vi "cblas ztrmm.vi"(0 "A":T2, 1 "B":T2, 3 "alpha":cdb=1.0+0.0i, 5 "order":T5=101 items=["CblasRowMajor"=101, "CblasColMajor"=102], 6 "transA":T6=111 items=["CblasNoTrans"=111, "CblasTrans"=112, "CblasConjTrans "=113], 7 "uplo":T4=121 items=["CblasUpper"=121, "CblasLower"=122], 8 "lda":i32, 9 "m":i32=-1, 10 "ldb":i32, 11 "n":i32=-1, 12 "diag":T3=131 items=["CblasNonUnit"=131, "CblasUnit"=132], 13 "side":T1=141 items=["CblasLeft"=141, "CblasRight"=142]) -> (14 "ztrmm":T2, 19 "error":i32)   [LabVIEW 2017, in "NI_AALBLAS.lvlib"]
uses:
  NI_AALBLAS.lvlib
  ComplexMatrix.ctl
  Operation_Transpose.ctl
  Order.ctl
  UpLo.ctl
  Diag.ctl
  Side.ctl
  <resource>/lvblas.dll
  NI_Matrix.lvlib
panel:
  # "void cblas_ztrmm(order, side, uplo, transA, diag, m, n, *alpha, *A, lda, *X, ldx)"
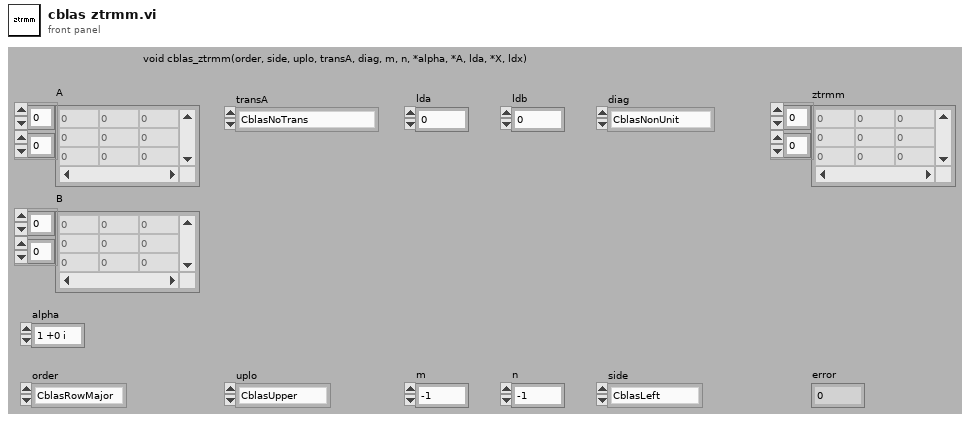
[diagram p1: front panel]
types:
  T1 = typedef "NI_AALBLAS.lvlib/Side.ctl" = i32
  T2 = typedef "NI_Matrix.lvlib/ComplexMatrix.ctl" = cdb[][]
  T3 = typedef "NI_AALBLAS.lvlib/Diag.ctl" = i32
  T4 = typedef "NI_AALBLAS.lvlib/UpLo.ctl" = i32
  T5 = typedef "NI_AALBLAS.lvlib/Order.ctl" = i32
  T6 = typedef "NI_AALBLAS.lvlib/Operation_Transpose.ctl" = i32
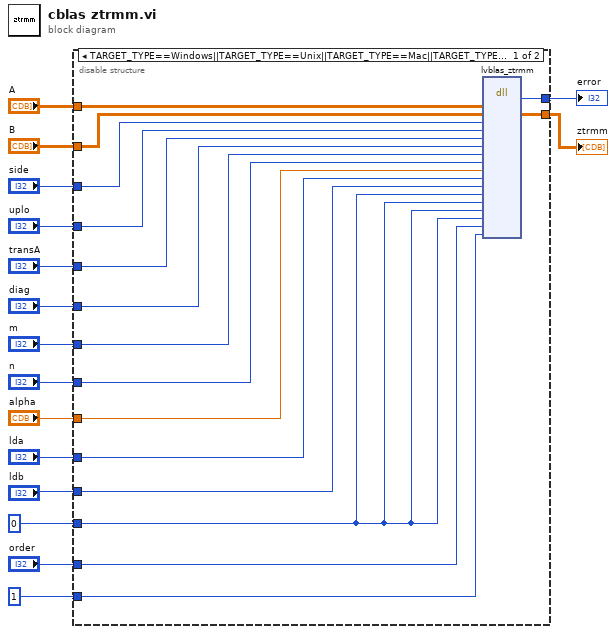
[diagram p0: block diagram]
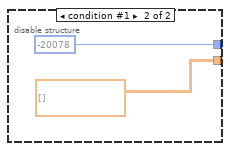
[diagram p2: hidden frame]
diagram:
  n1 = disable-structure shown="TARGET_TYPE==Windows||TARGET_TYPE==Unix||TARGET_TYPE==Mac||TARGET_TYPE==RT" {
    disable-tunnel: "A" -> [w32 _]
    disable-tunnel: [w31 -20078 ("error")] -> w15
    disable-tunnel: 0 -> [w23 _]
    disable-tunnel: [w30 cdb[][] [] ("y")] -> w7
    disable-tunnel: "transA" -> [w26 _]
    disable-tunnel: "uplo" -> [w27 _]
    disable-tunnel: "diag" -> [w25 _]
    disable-tunnel: "B" -> [w29 _]
    disable-tunnel: "side" -> [w28 _]
    disable-tunnel: "alpha" -> [w24 _]
    disable-tunnel: "order" -> [w22 _]
    disable-tunnel: "m" -> [w21 _]
    disable-tunnel: "n" -> [w20 _]
    disable-tunnel: "lda" -> [w19 _]
    disable-tunnel: "ldb" -> [w18 _]
    disable-tunnel: 1 -> [w17 _]
    frame condition #0 (active) {
      n2 = dll-call lib="C:/Program Files (x86)/National Instruments/LabVIEW 2017/resource/lvblas.*" fn="lvblas_ztrmm" ("CBLAS.dll:MtrxxVectH")("a"=w32, "x"=w29, "side"=w28, "uplo"=w27, "OpA"=w26, "diag"=w25, "m"=w21, "n"=w20, "alpha"=w24, "lda"=w19, "ldx"=w18, "startARow"=w23, "startACol"=w23, "startXRow"=w23, "startXCol"=w23, "order"=w22, "check"=w17) -> ("error"=w31:i32, "x"=w30:T2)  [unwired: 19 in, 2 out]
    }
    frame condition #1 {
    }
  }
  "ztrmm" <- w7
  "error" <- w15
